vi "trace_toLVBuffer_interferogram.vi"(0 "reference":refnum<class "OSA.lvclass">, 2 "idx latest":bool, 3 "trace idx interferogram":u32, 5 "error in (no error)":errorcluster) -> (14 "duplicate reference":refnum<class "OSA.lvclass">, 17 "trace length":u32, 19 "error out":errorcluster)   [LabVIEW 2010, in "OSA.lvclass"]
doc: "Reads data from trace buffer and updates labview allocated buffer specrtum Y array, X is equidistant and only x min and max are retrieved, or X are filled with an x-value for each y ditto. \n\nX: optical path length (cm)\nY: ADC value"
uses:
  OSA.lvclass
  typeDef/trace_properties_ui.ctl
  typeDef/trace_properties_double.ctl
  typeDef/acq_dataType.ctl
  FTSLib.dll
  OSA20X_misc.lvlib
panel:
  in  "property double":T1=enum."x_max"
  in  "property":T2
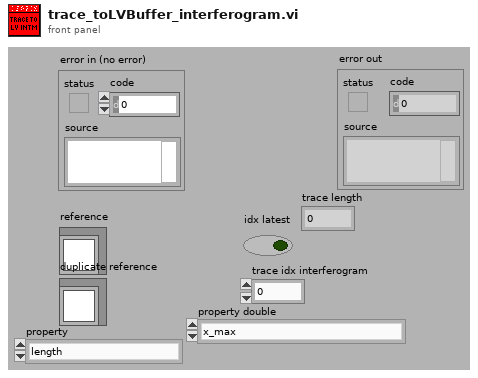
[diagram p1: front panel]
types:
  T1 = typedef "OSA.lvclass/trace_properties_double.ctl" = enum16{"x_minWnr", "x_maxWnr", "x_min", "x_max", "y_min", "y_max", "resolution", "referenceWavelength_nm_vac", "samplingDistance_cm_vac", "zeroFillFactor", "air_temp", "air_press", "air_relHum", "minOPD_cm", "maxOPD_cm", "interferogramOffset", "apodizationPowerCompensation", "integrationTime_ms", "gainLevel", "all_doubleProperties"}
  T2 = typedef "OSA.lvclass/trace_properties_ui.ctl" = enum16{"length", "type", "acquisitionMode", "xValueFormat", "date", "time", "averageNum", "smoothType", "igramSmoothType", "phaseCorrection", "apodisation", "__allocatedLengthI", "__allocatedLengthx", "adcBits", "sensitivityMode", "resolutionMode", "rollingAverage", "samplesPerReference", "air_measureOption", "interferogramProperty", "all_uiProperties"}
  T3 = typedef "OSA.lvclass/acq_dataType.ctl" = enum16{"none", "interferogram", "spectrum"}
  T4 = enum16{"get", "init", "set interferogram", "set spectrum", "cleanUp"}
  T5 = typedef "OSA.lvclass/ObjectAttributes.ctl" = cluster{"Stop":bool, "dataType":T3, "spectrometerIdx":u16, "buffer size interferogram":i32, "interferogram":cluster{"new":bool, "plot_x_ min":sgl, "plot_x_max":sgl, "plot_y_min":sgl, "plot_y_max":sgl, "Graph Intrfrgrm":T6, "timeStamp":u32, "signal (%)":dbl, "traces":cluster{"idx":u32, "broadBand":bool, "monoChromatic":bool, "peakToPeakSignal":dbl, "peakToPeakPos":dbl}[], "traces idx last":i32}, "spectrum":cluster{"new":bool, "plot_x_min":sgl, "plot_x_max":sgl, "plot_unit_x":T7, "plot_unit_y":T8, "plot_y_min":sgl, "plot_y_max":sgl, "Graph Spectrum":T6, "timeStamp":u32, "X_VAL_OPTIONS":enum16{"MIN_MAX", "ARRAY"}, "traces":cluster{"idx":u32}[], "traces idx last":i32}, "Thorlabs_OSA_64.lvclass:queue_action.ctlqueue ref":refnum<queue>, "action":T9, "plot zoom step":dbl, "buffer semaphore":T10, "acq stopped":bool, "dataType active":T3, "temperature (degr C)":sgl, "pressure (hPa)":sgl, "rel humidity (%)":sgl, "settings":cluster{"resolution":u16, "sensitivity":u16, "Average":bool, "average nr":u32, "apodisation":T11, "acq delay (ms)":u32, "airMesure":T12, "wmtr on":bool, "intfgrm_smooth_width":u16, "intfgrm_smooth_nrOfPasses":u16, "intfgrm_smooth":T13, "phaseCorrection":T14, "zeroFill":u8, "spectr_smooth":T13, "spectr_smooth_width":u16, "spectr_smooth_nrOfPasses":u16, "resolution (/cm)":sgl, "REF wavelength, (nm)":dbl, "gain_idx":u16, "gainAuto":bool, "gain_relative":dbl, "PD sensitivity mode":T15, "PD senseMode implemented":bool, "SensorTemperature implemented":bool, "SensorPressure implemented":bool, "SensorHumidity implemented":bool, "attenuationAuto":bool, "attenuationOnOff":bool, "attenuationAvailable":bool, "offsetAvailable":bool, "offset":i32, "offset max":u16}, "peaks position":sgl[], "peaks width":sgl[], "peaks height":sgl[], "peaks max nr":u32, "peaks latest nr":i32, "peaks new":bool, "power":dbl, "power new":bool, "path":string, "wavelength (WNr)":dbl, "wavelength new":bool, "buffer size spectrum":i32, "status":string, "VI reference":refnum<vi>, "funcPointer":u64, "libraryPointer":u64, "singleAcquisition":bool, "coherenceLength (cm)":dbl, "coherenceLength new":bool, "spectrometer model":string, "spectrometer serial nr":string, "peaks thld left":sgl[], "peaks thld right":sgl[], "coherenceLength error (cm)":dbl, "ADC bits":u16, "peaks position centroid":sgl[], "peaks height centroid":sgl[], "OSA series":T16, "channel index spectrum":u16, "spectrometer rangeLow, (/cm)":dbl, "spectrometer rangeHigh, (/cm)":dbl, "channel index interferogram":u16}
  T6 = typedef "OSA.lvclass/graph_intensity.ctl" = refnum<vi>
  T7 = typedef "OSA.lvclass/spectrum_x_unit.ctl" = enum16{"wavenr/cm", "THz", "eV", "nm_air", "nm_vac"}
  T8 = typedef "OSA.lvclass/y_unit.ctl" = enum16{"ADC counts", "dBm pwr absolute", "dBm pwr density", "mW pwr absolute", "mW pwr density"}
  T9 = typedef "OSA.lvclass/queue_action.ctl" = enum16{"none", "stop", "GUI_plotInterferogram", "GUI_plotSpectrum", "GUI_plotInterferogramRescale", "GUI_plotSpectrumRescale", "GUI_plotInterferogramReset", "GUI_plotSpectrumReset", "GUI_plotInterferogramAutoScaleY", "GUI_plotSpectrumAutoScaleY", "GUI_plotInterferogramZoomOut", "GUI_plotSpectrumZoomOut", "GUI_plotInterferogramPane", "GUI_plotSpectrumPane", "GUI_plotInterferogramZoomMouse", "GUI_plotSpectrumZoomMouse", "GUI_spectrumChannelType", "GUI_channel", "ENVIRONMENT temperature", "ENVIRONMENT pressure", "MODE_resolution set", "MODE_resolution get", "MODE_sensitivity set", "MODE_sensitivity get", "MODE_PDTemperature set", "MODE_PDTemperature get", "REBOOT/RESET firmware", "ACQASYNC_acquireSingleSpectrum", "ACQASYNC_continuous start", "ACQASYNC_continuous stop\n", "ACQASYNC_get last interferogram", "ACQASYNC_get last spectrum", "ACQASYNC_get last waveNr", "ACQOPT_interferogram smoothing set", "ACQOPT_interferogram smoothing get", "ACQOPT_spectrum smoothing set", "ACQOPT_spectrum smoothing get", "ACQOPT_apodisation type set", "ACQOPT_apodisation type get", "ACQOPT_phase correction type set", "ACQOPT_phase correction type get", "ACQOPT_acqIntervall_set", "ACQOPT_acqIntervall_get", "ACQOPT_average spectrum set", "ACQOPT_average spectrum get", "ACQOPT_rolling average set", "ACQOPT_rolling average get", "ACQOPT_zero fill factor set", "ACQOPT_zero fill factor get", "ACQOPT_cycle counting set", "ACQOPT_cycle counting get", "ACQOPT_air measure option set", "ACQOPT_air measure option get", "ACQOPT_gainLevel auto get", "ACQOPT_gainLevel auto set", "ACQOPT_gainLevel get", "ACQOPT_gainLevel set", "ACQOPT_getAll", "INSTRUMENT_PROPERTY_range_WaveNr_min", "INSTRUMENT_PROPERTY_range_WaveNr_max", "INSTRUMENT_PROPERTY_reference_wavelength_cm^-1", "INSTRUMENT_PROPERTY_samplesPerRefPeriod", "INSTRUMENT_PROPERTY_resolution_waveNrPercm", "INSTRUMENT_PROPERTY_availableGainLevels", "INSTRUMENT_PROPERTY_status", "CONVERT", "ANALYSE_POWER", "ANALYSE_PEAKS", "ANALYSE_WAVELENGTH", "ANALYSE_SPECTRUM", "ANALYSE_INTERFEROGRAM", "ANALYSE_COHERENCE_LENGTH", "MATH", "MATH_power", "MATH_peaks", "FILE", "miscellaneous"}
  T10 = typedef "Semaphore RefNum" = refnum<k1>
  T11 = typedef "OSA.lvclass/apodisation.ctl" = enum16{"NONE", "NORTON_BEER_WEAK", "NORTON_BEER_MEDIUM", "NORTON_BEER_STRONG", "TRIANGULAR", "COSINE", "HANN", "HAMMING", "BLACKMANHARRIS3", "BLACKMANHARRIS4", "GAUSSIAN"}
  T12 = typedef "OSA.lvclass/airMeasure.ctl" = enum16{"TEMPERATURE", "PRESSURE"}
  T13 = typedef "OSA20X_misc.lvlib/interferogram_smoothing.ctl" = enum16{"NONE", "BINOMIAL", "SAVITSKY_GOLAY", "FOURIER", "MOVING_AVERAGE", "GAUSSIAN"}
  T14 = typedef "OSA.lvclass/phaseCorrection.ctl" = enum16{"NONE", "MERTZ", "FORMAN", "MERTZ_FILE", "FORMAN_FILE", "FUTURE COMP."}
  T15 = typedef "OSA20X_misc.lvlib/PDTemperatureMode.ctl" = enum16{"cool: better sensitivity/noise floor", "warm: extended wl range"}
  T16 = typedef "OSA.lvclass/OSA_series.ctl" = enum16{"OSA200", "OSA300", "UNKNOWN"}
  T17 = cluster{"length":u32, "X min (cm)":sgl, "X max (cm)":sgl, "saturated":bool, "broadband":bool, "isMonoChromatic":bool, "peakToPeak, (counts)":dbl, "peakToPeak position (cm)":dbl, "samplesPerRefPeriod":i32}
  T18 = cluster{"idx":u32, "broadBand":bool, "monoChromatic":bool, "peakToPeakSignal":dbl, "peakToPeakPos":dbl}[]
  T19 = cluster{"idx":u32, "broadBand":bool, "monoChromatic":bool, "peakToPeakSignal":dbl, "peakToPeakPos":dbl}
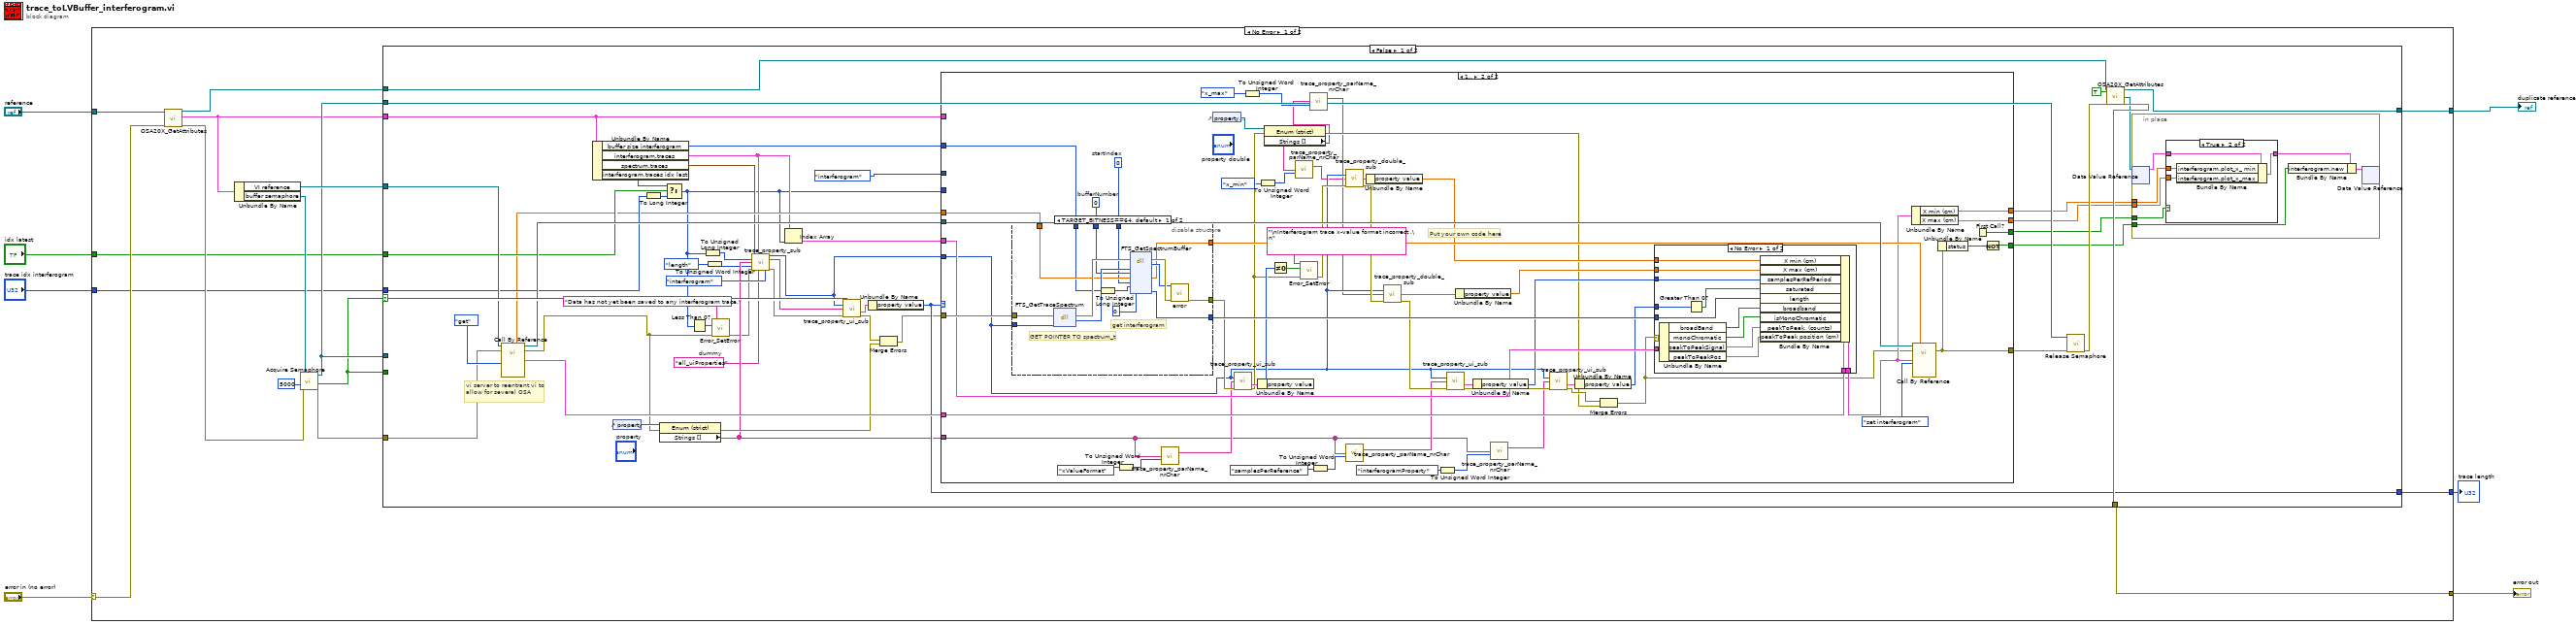
[diagram p0: block diagram]
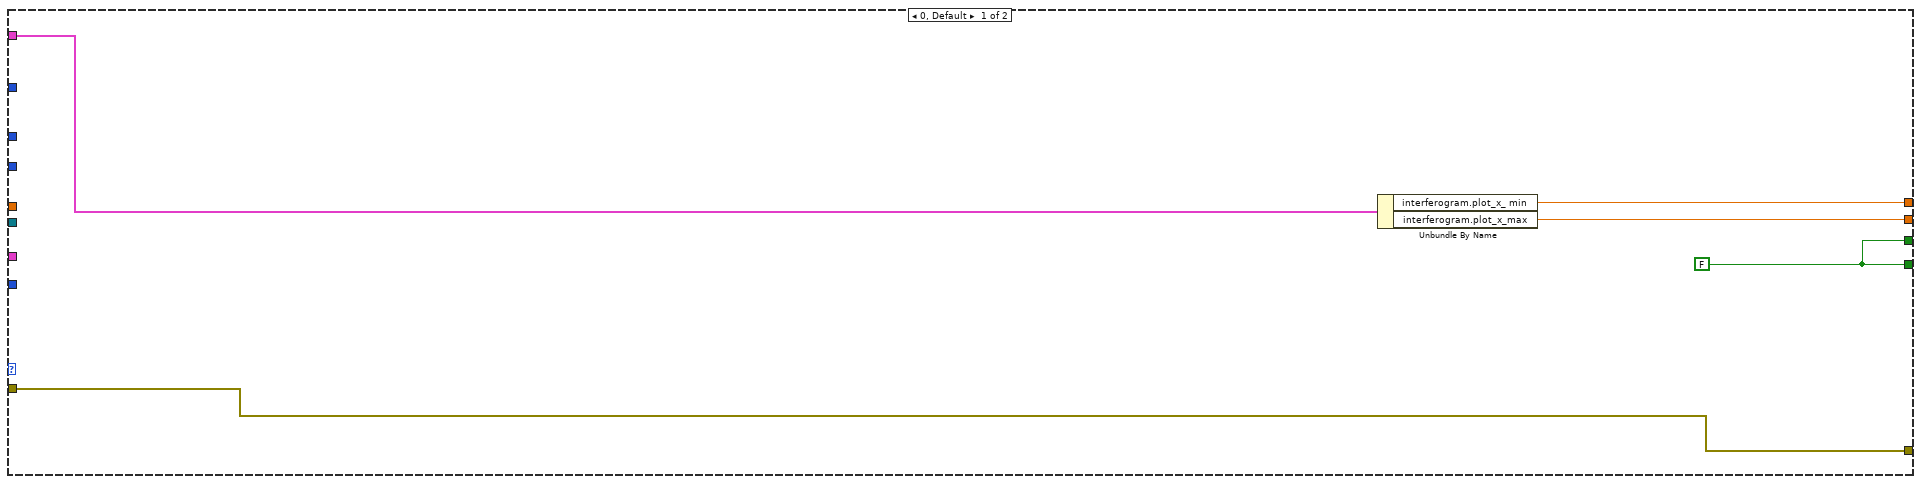
[diagram p2: hidden frame]
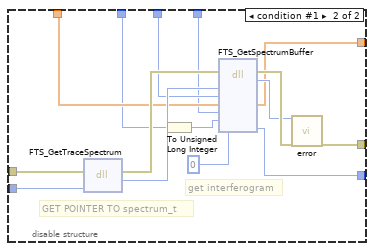
[diagram p4: hidden frame]
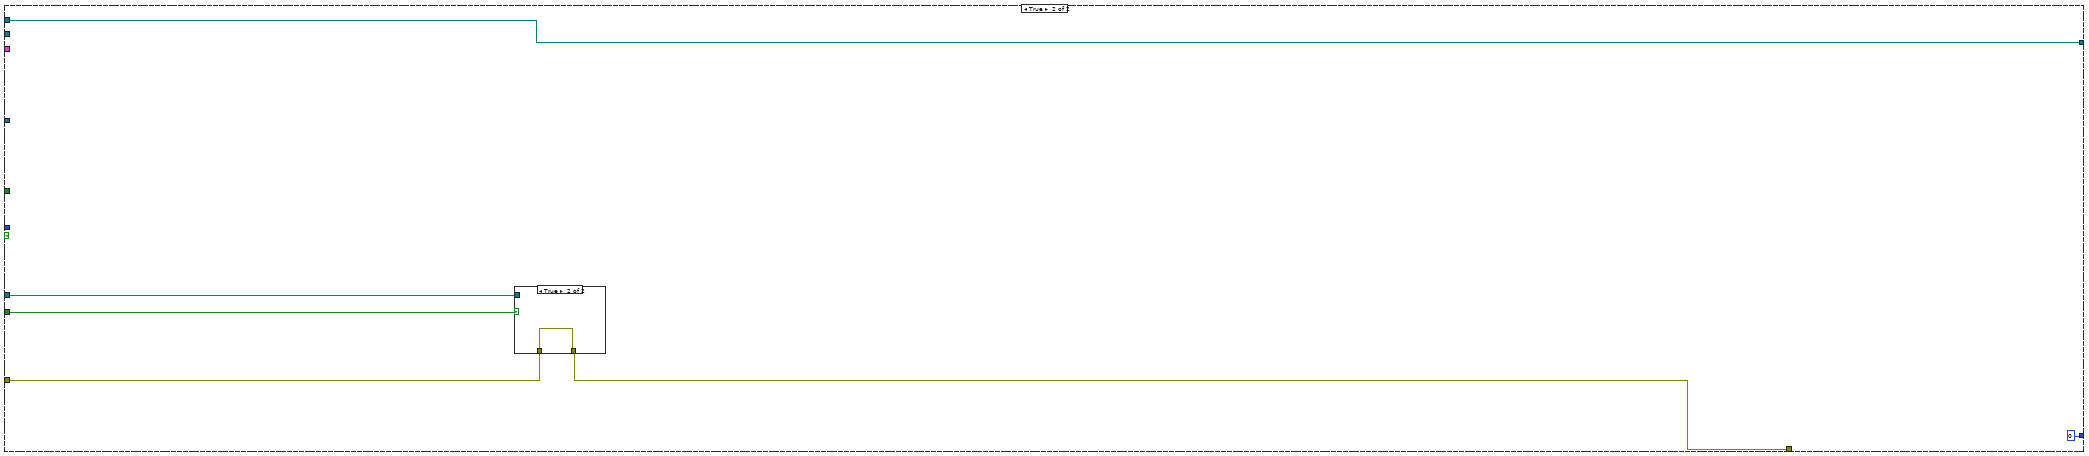
[diagram p6: hidden frame]
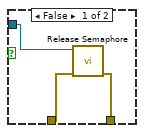
[diagram p7: hidden frame]
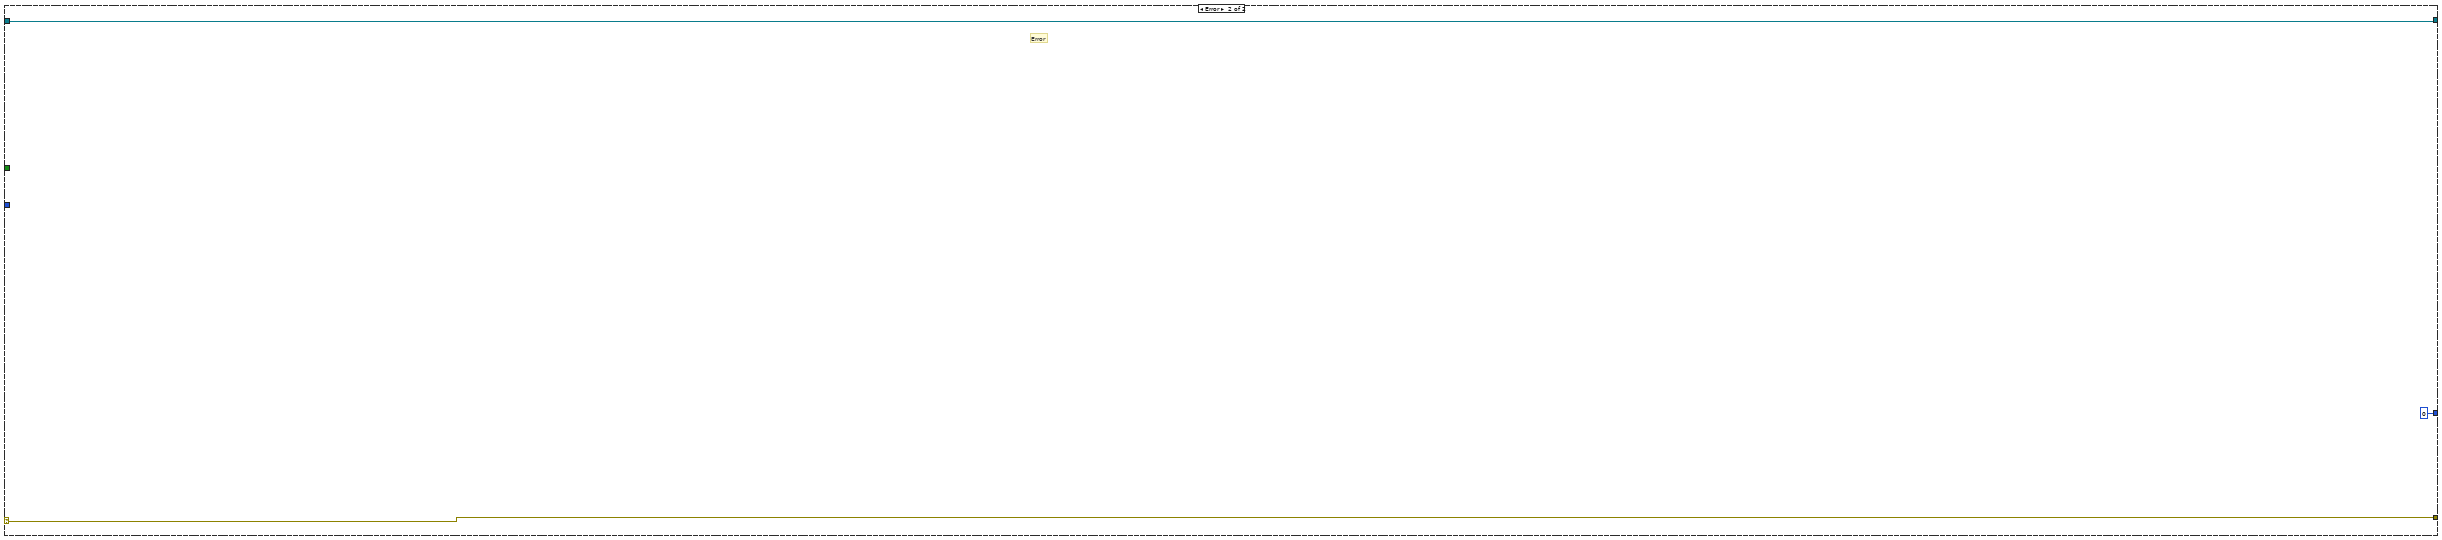
[diagram p8: hidden frame]
diagram:
  n1 = case shown="No Error" "error in (no error)" {
    selector: "error in (no error)" -> [w22 w203]
    tunnel: [w21 w203] -> w6
    tunnel: "reference" -> [w23 w202]
    tunnel: [w20 w202] -> w4
    tunnel: "idx latest" -> [w11 _]
    tunnel: "trace idx interferogram" -> [w10 _]
    tunnel: [w9 u32 0 ("property value")] -> w1
    frame No Error {
      n2 = call "OSA20X_GetAttributes.vi"("reference in"=w23, "error in (no error)"=w22) -> ("reference out"=w14:refnum<class "OSA.lvclass">, "Data"=w12:T5, "error out"=w18:errorcluster)  [unwired: 14 in, 1 out]
      n3 = Unbundle By Name(w12) -> ("VI reference"=w15:refnum<vi>, "buffer semaphore"=w19:T10)
      n4 = call <vilib>:"Acquire Semaphore.vi"("error in (no error)"=w18, "ms timeout (-1)"=5000, "semaphore"=w19) -> ("error out"=w16:errorcluster, "timed out"=w8:bool, "semaphore out"=w13:T10)  [unwired: 2 in]
      n5 = case shown="False" w8 {
        tunnel: w12 -> [w48 _]
        tunnel: w16 -> [w65 w193]
        tunnel: [w71 w192] -> w21
        tunnel: [w70 w196] -> w20
        tunnel: w13 -> [w67 _]
        tunnel: w15 -> [w64 _]
        tunnel: w14 -> [w38 w196]
        tunnel: w8 -> [_ w195]
        tunnel: w13 -> [_ w194]
        tunnel: w11 -> [w60 _]
        tunnel: w10 -> [w58 _]
        tunnel: [w46 u32 0 ("property value")] -> w9
        frame False {
          w24 = "all_uiProperties"  # dummy
          # "vi server to reentrant vi to \nallow for several OSA"
          n6 = call-by-ref "?"(reference=w64, error in=w65, "action"=T4."get") -> (reference out=w63:refnum<vi>, error out=w42:errorcluster, "interferogram"=w54:sgl[], "interferogram prop set"=w52:T17)  [unwired: 14 in, 3 out]
          n7 = Unbundle By Name(w48) -> ("buffer size interferogram"=w53:i32, "interferogram.traces"=w37:T18, "spectrum.traces"=w36:cluster{"idx":u32}[], "interferogram.traces idx last"=w59:i32)
          n8 = control-ref of="property"() -> (w43:refnum<vi>)
          n9 = To Long Integer(number=w58) -> (32bit integer=w57:i32)
          n10 = property class="Enum (strict)"(reference=w43, error in=w42) -> (error out=w39:errorcluster, "Strings []"=w32:string[])  [unwired: 1 out]
          n11 = Select(t=w59, s=w60, f=w57) -> (s? t:f=w26:i32)
          n12 = Less Than 0?(x=w26) -> (x < 0?=w56:bool)
          n13 = To Unsigned Long Integer(number=w26) -> (unsigned 32bit integer=w25:u32)
          n14 = To Unsigned Word Integer(number=trace_properties_ui."length" ("property")) -> (unsigned 16bit integer=w27:u16)
          n15 = call "Error_SetError.vi"("error in"=w42, "status (true)"=w56, "source(\"\")"="Data has not yet been saved to any interferogram trace." ("source(\"\")")) -> ("error out"=w31:errorcluster)  [unwired: 4 in]
          n16 = call "trace_property_sub.vi"("traces_spectrum"=w36, "traces_interferogram"=w37, "trace idx"=w25, "Strings enum"=w32, "Value enum"=w27, "error in (no error)"=w31, "all string"=w24, "dataType"=acq_dataType."interferogram") -> ("global trace idx"=w34:u32, "parameter names"=w33:string[], "error out"=w30:errorcluster)  [unwired: 4 in, 1 out]
          n17 = Index Array(array=w37, index=w26) -> (element=w40:T19)
          n18 = call "trace_property_ui_sub.vi"("trace idx global"=w34, "properties ui"=w33, "error in (no error)"=w30) -> ("property"=w41:cluster{"property":string, "property value":u32}, "error out"=w29:errorcluster)  [unwired: 10 in, 1 out]
          n19 = Unbundle By Name(w41) -> ("property value"=w46:u32)
          n20 = Merge Errors(w29, w39) -> (w28:errorcluster)
          n21 = case shown="1.." w46 {
            tunnel: [w73 w122] -> w68
            tunnel: w63 -> [_ w133]
            tunnel: w54 -> [_ w132]
            tunnel: w53 -> [_ w131]
            tunnel: w52 -> [_ w130]
            tunnel: [w75 w127] -> w51
            tunnel: [w74 w126] -> w50
            tunnel: w26 -> [_ _]
            tunnel: w28 -> [w73 w123]
            tunnel: [w72 w120] -> w49
            tunnel: w48 -> [w76 _]
            tunnel: acq_dataType."interferogram" ("dataType") -> [_ _]
            tunnel: [w72 w115] -> w45
            tunnel: w40 -> [_ w114]
            tunnel: w34 -> [_ w89]
            tunnel: w32 -> [_ w84]
            frame 0, Default {
              w72 = FALSE
              n22 = Unbundle By Name(w76) -> ("interferogram.plot_x_ min"=w75:sgl, "interferogram.plot_x_max"=w74:sgl)
            }
            frame 1.. {
              w124 = u32 0  # startIndex
              w125 = 0  # bufferNumber
              # "Put your own code here"
              n23 = disable-structure shown="TARGET_BITNESS==64, default" {
                disable-tunnel: w123 -> [w162 w166]
                disable-tunnel: [w149 w164] -> w112
                disable-tunnel: w89 -> [w163 w165]
                disable-tunnel: w132 -> [w159 w170]
                disable-tunnel: w131 -> [w158 w169]
                disable-tunnel: [w153 w172] -> w129
                disable-tunnel: [w152 w171] -> w128
                disable-tunnel: w125 -> [w151 w168]
                disable-tunnel: w124 -> [w150 w167]
                frame condition #0 (active) {
                  # "get interferogram"
                  # "GET POINTER TO spectrum_t"
                  n24 = dll-call lib="FTSLib.dll" fn="FTS_GetTraceSpectrum"(error in=w162, "traceIdx"=w163) -> (error out=w161:errorcluster, "spectrum_t_pointer"=w160:u64)  [unwired: 3 in, 1 out]
                  n25 = To Unsigned Long Integer(number=w158) -> (unsigned 32bit integer=w157:u32)
                  n26 = dll-call lib="FTSLib.dll" fn="FTS_GetSpectrumBuffer"(error in=w161, "source"=w160, "bufferNumber"=w151, "destination"=w159, "startIndex"=w150, "length"=w157, "vaulesCopied"=u32 0) -> (error out=w155:errorcluster, "return type"=w154:i32, "destination"=w152:sgl[], "vaulesCopied"=w153:u32)  [unwired: 6 in, 1 out]
                  n27 = call "error.vi"("result code"=w154, "error in (no error)"=w155) -> ("error out"=w149:errorcluster)  [unwired: 15 in, 2 out]
                }
                frame condition #1 {
                  # "get interferogram"
                  # "GET POINTER TO spectrum_t"
                  n28 = dll-call lib="FTSLib.dll" fn="FTS_GetTraceSpectrum"(error in=w166, "traceIdx"=w165) -> (error out=w178:errorcluster, "spectrum_t_pointer"=w177:u32)  [unwired: 3 in, 1 out]
                  n29 = To Unsigned Long Integer(number=w169) -> (unsigned 32bit integer=w176:u32)
                  n30 = dll-call lib="FTSLib.dll" fn="FTS_GetSpectrumBuffer"(error in=w178, "source"=w177, "bufferNumber"=w168, "destination"=w170, "startIndex"=w167, "length"=w176, "vaulesCopied"=u32 0) -> (error out=w174:errorcluster, "return type"=w173:i32, "destination"=w171:sgl[], "vaulesCopied"=w172:u32)  [unwired: 6 in, 1 out]
                  n31 = call "error.vi"("result code"=w173, "error in (no error)"=w174) -> ("error out"=w164:errorcluster)  [unwired: 15 in, 2 out]
                }
              }
              n32 = To Unsigned Word Integer(number=trace_properties_ui."xValueFormat" ("property")) -> (unsigned 16bit integer=w88:u16)
              n33 = call "trace_property_parName_nrChar.vi"("Strings enum"=w84, "Value enum"=w88) -> ("parameter names"=w87:string[])  [unwired: 12 in, 1 out]
              n34 = control-ref of="property double"() -> (w102:refnum<vi>)
              n35 = call "trace_property_ui_sub.vi"("trace idx global"=w89, "properties ui"=w87, "error in (no error)"=w112) -> ("property"=w111:cluster{"property":string, "property value":u32}, "error out"=w101:errorcluster)  [unwired: 10 in, 1 out]
              n36 = To Unsigned Word Integer(number=trace_properties_double."x_max" ("property")) -> (unsigned 16bit integer=w81:u16)
              n37 = Unbundle By Name(w111) -> ("property value"=w110:u32)
              n38 = To Unsigned Word Integer(number=trace_properties_double."x_min" ("property")) -> (unsigned 16bit integer=w79:u16)
              n39 = property class="Enum (strict)"(reference=w102, error in=w101) -> (error out=w91:errorcluster, "Strings []"=w78:string[])  [unwired: 1 out]
              n40 = Not Equal To 0?(x=w110) -> (x != 0?=w118:bool)
              n41 = call "trace_property_parName_nrChar.vi"("Strings enum"=w78, "Value enum"=w79) -> ("parameter names"=w77:string[])  [unwired: 12 in, 1 out]
              n42 = call "Error_SetError.vi"("error in"=w101, "status (true)"=w118, "source(\"\")"="\nInterferogram trace x-value format incorrect .\n" ("source(\"\")")) -> ("error out"=w97:errorcluster)  [unwired: 4 in]
              n43 = call "trace_property_parName_nrChar.vi"("Strings enum"=w78, "Value enum"=w81) -> ("parameter names"=w80:string[])  [unwired: 12 in, 1 out]
              n44 = To Unsigned Word Integer(number=trace_properties_ui."samplesPerReference" ("property")) -> (unsigned 16bit integer=w86:u16)
              n45 = call "trace_property_double_sub.vi"("trace idx global"=w89, "properties ui"=w77, "error in (no error)"=w97) -> ("property"=w99:cluster{"property":string, "property value":dbl}, "error out"=w96:errorcluster)  [unwired: 10 in, 1 out]
              n46 = call "trace_property_parName_nrChar.vi"("Strings enum"=w84, "Value enum"=w86) -> ("parameter names"=w85:string[])  [unwired: 12 in, 1 out]
              n47 = Unbundle By Name(w99) -> ("property value"=w98:dbl)
              n48 = call "trace_property_double_sub.vi"("trace idx global"=w89, "properties ui"=w80, "error in (no error)"=w96) -> ("property"=w94:cluster{"property":string, "property value":dbl}, "error out"=w95:errorcluster)  [unwired: 10 in, 1 out]
              n49 = To Unsigned Word Integer(number=trace_properties_ui."interferogramProperty" ("property")) -> (unsigned 16bit integer=w83:u16)
              n50 = call "trace_property_ui_sub.vi"("trace idx global"=w89, "properties ui"=w85, "error in (no error)"=w95) -> ("property"=w107:cluster{"property":string, "property value":u32}, "error out"=w104:errorcluster)  [unwired: 10 in, 1 out]
              n51 = Unbundle By Name(w94) -> ("property value"=w117:dbl)
              n52 = Unbundle By Name(w107) -> ("property value"=w106:u32)
              n53 = call "trace_property_parName_nrChar.vi"("Strings enum"=w84, "Value enum"=w83) -> ("parameter names"=w82:string[])  [unwired: 12 in, 1 out]
              n54 = call "trace_property_ui_sub.vi"("trace idx global"=w89, "properties ui"=w82, "error in (no error)"=w104) -> ("property"=w105:cluster{"property":string, "property value":u32}, "error out"=w92:errorcluster)  [unwired: 10 in, 1 out]
              n55 = Unbundle By Name(w105) -> ("property value"=w103:u32)
              n56 = Merge Errors(w92, w91) -> (w90:errorcluster)
              n57 = case shown="No Error" w90 {
                tunnel: w130 -> [w147 w148]
                tunnel: w129 -> [w146 _]
                tunnel: [w145 w148] -> w116
                tunnel: w114 -> [w144 _]
                tunnel: w98 -> [w138 _]
                tunnel: w117 -> [w137 _]
                tunnel: w103 -> [w140 _]
                tunnel: w106 -> [w141 _]
                frame No Error {
                  n58 = Unbundle By Name(w144) -> ("broadBand"=w136:bool, "monoChromatic"=w135:bool, "peakToPeakSignal"=w143:dbl, "peakToPeakPos"=w142:dbl)
                  n59 = Greater Than 0?(x=w140) -> (x > 0?=w139:bool)
                  n60 = Bundle By Name(cluster=w147, "X min (cm)"=w138, "X max (cm)"=w137, "samplesPerRefPeriod"=w141, "saturated"=w139, "length"=w146, "broadband"=w136, "isMonoChromatic"=w135, "peakToPeak, (counts)"=w143, "peakToPeak position (cm)"=w142) -> (w145:T17)
                }
                frame Error {
                }
              }
              n61 = Unbundle By Name(w116) -> ("X min (cm)"=w127:sgl, "X max (cm)"=w126:sgl)
              n62 = call-by-ref "?"(reference=w133, error in=w90, "interferogram prop set"=w116, "action"=T4."set interferogram", "interferogram set"=w128) -> (error out=w122:errorcluster)  [unwired: 12 in, 6 out]
              n63 = Unbundle By Name(w122) -> ("status"=w121:bool)
              n64 = First Call?() -> (First Call?: T/F=w115:bool)
              n65 = Not(x=w121) -> (.not. x?=w120:bool)
            }
          }
          n66 = call <vilib>:"Release Semaphore.vi"("error in (no error)"=w68, "semaphore"=w67) -> ("error out"=w69:errorcluster)  [unwired: 4 in, 1 out]
          n67 = call "OSA20X_GetAttributes.vi"("reference in"=w38, "OnlyGetDvrReference(False)"=TRUE, "error in (no error)"=w69) -> ("reference out"=w70:refnum<class "OSA.lvclass">, "DataRef"=w61:refnum<data-value>, "error out"=w71:errorcluster)  [unwired: 13 in, 1 out]
          n68 = in-place {
            in-place-border: w45 -> [w185]
            in-place-border: w51 -> [w183]
            in-place-border: w50 -> [w182]
            in-place-border: w49 -> [w180]
            n69 = in-place-dvr #1(w61) -> (w184:T5)  [unwired: 1 out]
            n70 = case shown="True" w185 {
              tunnel: w184 -> [w186 w190]
              tunnel: [w186 w189] -> w181
              tunnel: w183 -> [_ w188]
              tunnel: w182 -> [_ w187]
              frame False {
              }
              frame True {
                n71 = Bundle By Name(cluster=w190, "interferogram.plot_x_ min"=w188, "interferogram.plot_x_max"=w187) -> (w189:T5)
              }
            }
            n72 = Bundle By Name(cluster=w181, "interferogram.new"=w180) -> (w179:T5)
            n73 = in-place-dvr #1(w179) -> ()  [unwired: 2 out]
          }
        }
        frame True {
          n74 = case shown="True" w195 {
            tunnel: w194 -> [w199 _]
            tunnel: w193 -> [w198 w200]
            tunnel: [w197 w200] -> w192
            frame False {
              n75 = call <vilib>:"Release Semaphore.vi"("error in (no error)"=w198, "semaphore"=w199) -> ("error out"=w197:errorcluster)  [unwired: 4 in, 1 out]
            }
            frame True {
            }
          }
        }
      }
    }
    frame Error {
      # "Error"
    }
  }
  "error out" <- w6
  "duplicate reference" <- w4
  "trace length" <- w1
